vi "write config ini data.vi"(8 "error in (no error)":errorcluster, 10 "data in":T2={"sections"=[], "key names"=[], "values"=[]}, 11 "Refnum in":T1) -> (0 "error out":errorcluster, 3 "Refnum out":T1)   [LabVIEW 2024, in "API Config Files Management.lvlib"]
doc: "This function writes the complete data from the input cluster to a configuration .ini file, regardless of the number of sections or the number of keys in each section. The input is a cluster containing three string arrays: a 2-D array for the sections, where the first row stores the section names and the second row contains the number of keys in each section; a 1-D string array for the key names; and a 1-D string array for the corresponding values."
uses:
  API Config Files Management.lvlib
  <vilib>/Utility/config.llb/NI_LVConfig.lvlib
  <vilib>/Utility/config.llb/Write Key (String).vi
  <vilib>/Utility/config.llb/Config Data RefNum.ctl
  config data.ctl
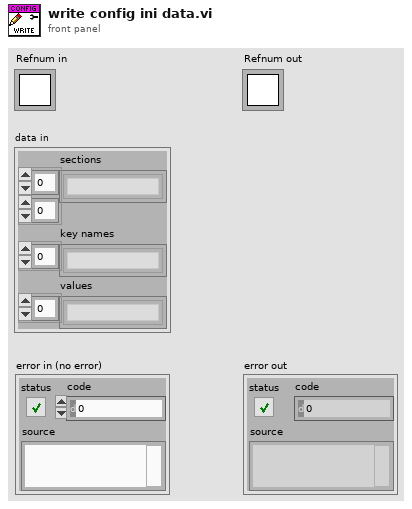
[diagram p1: front panel]
types:
  T1 = typedef "NI_LVConfig.lvlib/Config Data RefNum.ctl" = refnum<k1>
  T2 = typedef "config data.ctl" = cluster{"sections":string[][], "key names":string[], "values":string[]}
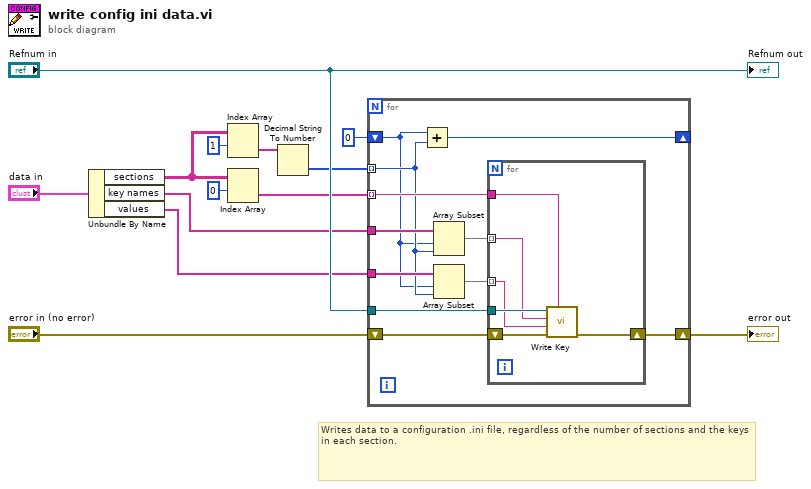
[diagram p0: block diagram]
diagram:
  # "Writes data to a configuration .ini file, regardless of the number of sections and the keys in each section."
  n1 = Unbundle By Name("data in") -> ("sections"=w9:string[][], "key names"=w11:string[], "values"=w10:string[])
  n2 = Index Array(array=w9, index (row)=1) -> (element=w5:string[])  [unwired: 1 in]
  n3 = Index Array(array=w9, index (row)=0) -> (element=w7:string[])  [unwired: 1 in]
  n4 = Decimal String To Number(string=w5) -> (number=w4:i32[])  [unwired: 2 in, 1 out]
  n5 = for {
    tunnel: w10 -> [w17]
    tunnel: w11 -> [w20]
    tunnel: "Refnum in" -> [w23]
    tunnel: w7 -> [w22] mode=indexing
    shift-right: [w21] -> w2
    shift-left: "error in (no error)" -> [w24]
    tunnel: w4 -> [w15] mode=indexing
    shift-right: [w18] -> _
    shift-left: 0 ("sector") -> [w14]
    n6 = Add(x=w14, y=w15) -> (x+y=w18:i32)
    n7 = Array Subset(array=w20, index=w14, length=w15) -> (w19:string[])
    n8 = Array Subset(array=w17, index=w14, length=w15) -> (w16:string[])
    n9 = for {
      tunnel: w23 -> [w30]
      shift-right: [w25] -> w21
      shift-left: w24 -> [w29]
      tunnel: w22 -> [w28]
      tunnel: w19 -> [w27] mode=indexing
      tunnel: w16 -> [w26] mode=indexing
      n10 = call-poly <vilib>:"Write Key.vi"("section"=w28, "error in (no error)"=w29, "value"=w26, "key"=w27, "refnum"=w30) -> ("error out"=w25:errorcluster)  [unwired: 4 in, 2 out]
    }
  }
  "error out" <- w2
  "Refnum out" <- "Refnum in"
